vi "Scan end Mode.vi"(8 "error in (no error)":errorcluster, 10 "Scan End Mode (Def: Stop)":enum16{"Stop", "Start"}(ring), 11 "VISA resource name":refnum<visa-resource-name>) -> (0 "error out":errorcluster, 3 "VISA resource name out":refnum<visa-resource-name>)   [LabVIEW 2015, in "SR400.lvlib"]
doc: "NE { j }\nIf j = 0, the NE command sets the scan end mode\n(AT N) to STOP. If j = 1, the mode is set to\nSTART. The scan end mode may be changed at\nany time. If j is absent, the scan end mode is\nreturned."
uses:
  SR400.lvlib
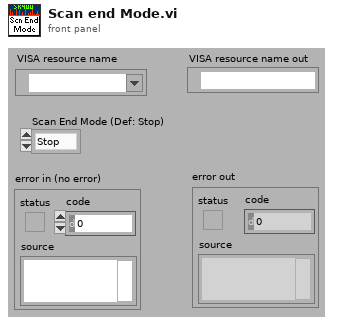
[diagram p1: front panel]
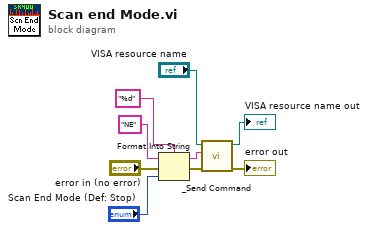
[diagram p0: block diagram]
diagram:
  n1 = Format Into String(format string="%d", initial string="NE" ("command"), error in="error in (no error)", "Scan End Mode (Def: Stop)") -> (resulting string=w5:string, error out=w4:errorcluster)
  n2 = call "_Send Command.vi"("error in (no error)"=w4, "Command"=w5, "VISA resource name"="VISA resource name") -> ("error out"=→"error out":errorcluster, "VISA resource name out"=→"VISA resource name out":refnum<visa-resource-name>)  [unwired: 1 in, 6 out]
